vi "how_many_indentation.vi"(11 "input":string) -> (2 "indentation":string, 3 "remain":string)   [LabVIEW 2019, in "User lib.lvlib"]
uses:
  User lib.lvlib
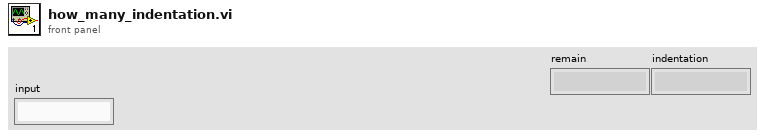
[diagram p1: front panel]
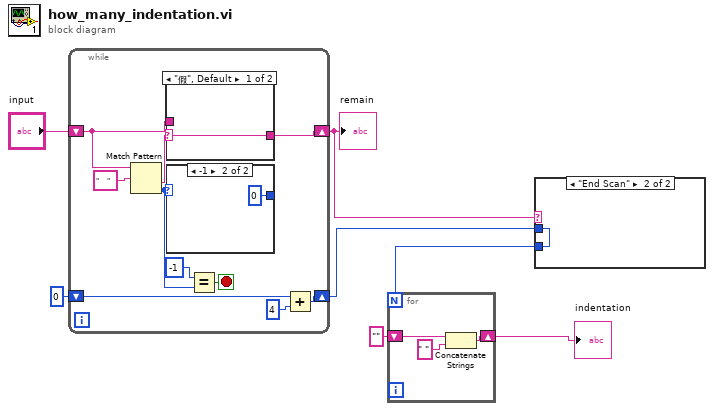
[diagram p0: block diagram]
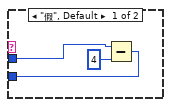
[diagram p2: hidden frame]
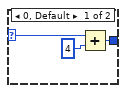
[diagram p4: hidden frame]
diagram:
  n1 = while {
    shift-right: [w11] -> w3
    shift-left: 0 ("offset past match") -> [w13]
    shift-right: [w8] -> w4
    shift-left: "input" -> [w9]
    stop <- w16 stop-if-true
    n2 = Match Pattern(string=w9, regular expression="    " ("正则表达式")) -> (after substring=w10:string, offset past match=w14:i32)  [unwired: 1 in, 2 out]
    n3 = case shown="\"假\", Default" w10 {
      selector: w10 -> [w18 _]
      tunnel: w9 -> [_ w19]
      tunnel: [w18 w19] -> w8
      frame "假", Default {
      }
      frame "" {
      }
    }
    n4 = case shown="-1" w14 {
      selector: w14 -> [w22 _]
      tunnel: [w20 0 ("offset past match")] -> _
      frame 0, Default {
        n5 = Add(x=w22, y=4) -> (x+y=w20:i32)
      }
      frame -1 {
      }
    }
    n6 = Equal?(x=-1, y=w14) -> (x = y?=w16:bool)
    n7 = Add(x=w13, y=4) -> (x+y=w11:i32)
  }
  "remain" <- w4
  n8 = case shown="\"End Scan\"" w4 {
    tunnel: w3 -> [w25 w27]
    tunnel: [w24 w27] -> w2
    frame "假", Default {
      n9 = Subtract(x=w25, y=4) -> (x-y=w24:i32)
    }
    frame "End Scan" {
    }
  }
  n10 = for {
    N: w2 -> [_]
    shift-right: [w29] -> w1
    shift-left: "" -> [w28]
    n11 = Concatenate Strings(w28, " ") -> (w29:string)
  }
  "indentation" <- w1
